vi "GFITS_VAR_postImgScript.vi"(5 "script name in":string, 7 "action":enum16{"read", "write"}(ring)) -> (8 "script name out":string)   [LabVIEW 2016]
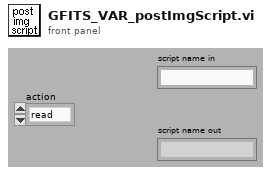
[diagram p1: front panel]
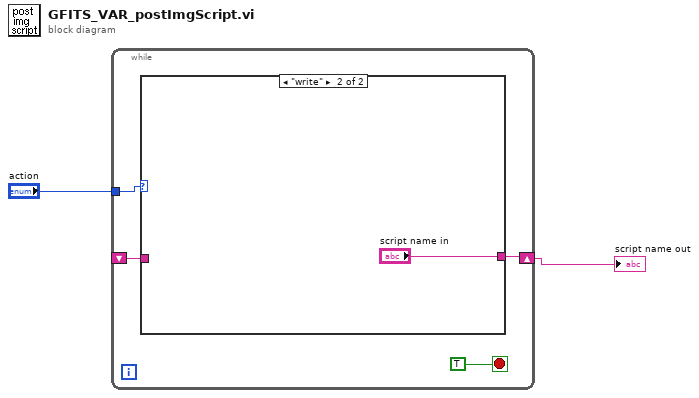
[diagram p0: block diagram]
diagram:
  n1 = while {
    tunnel: "action" -> [w5]
    shift-right: [w4] -> w1
    shift-left: _ -> [w3]
    stop <- TRUE stop-if-true
    n2 = case shown="\"write\"" w5 {
      tunnel: [w7 "script name in"] -> w4
      tunnel: w3 -> [w7 _]
      frame "read", Default {
      }
      frame "write" {
      }
    }
  }
  "script name out" <- w1
